vi "Acroname_Port_Enable.vi"(8 "error in (no error)":errorcluster, 9 "Current Max Amps limit (1.2)":dbl=1.2 format="%#_13g", 11 "Port Number":i32) -> (0 "error out":errorcluster, 1 "Max Current (µA)":u32, 2 "Min Voltage (µV)":u32, 3 "Enable Successful?":bool)   [LabVIEW 2025]
uses:
  1b1786e0-183b-4c19-b690-1d9e1fdb2131.vi
  27beaf38-548c-40ef-8c97-2fa24fe30fbd.vi
  31bf49dc-6773-40db-bb53-a572b45535a5.vi
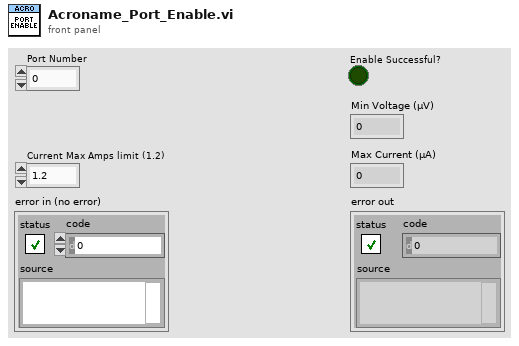
[diagram p1: front panel]
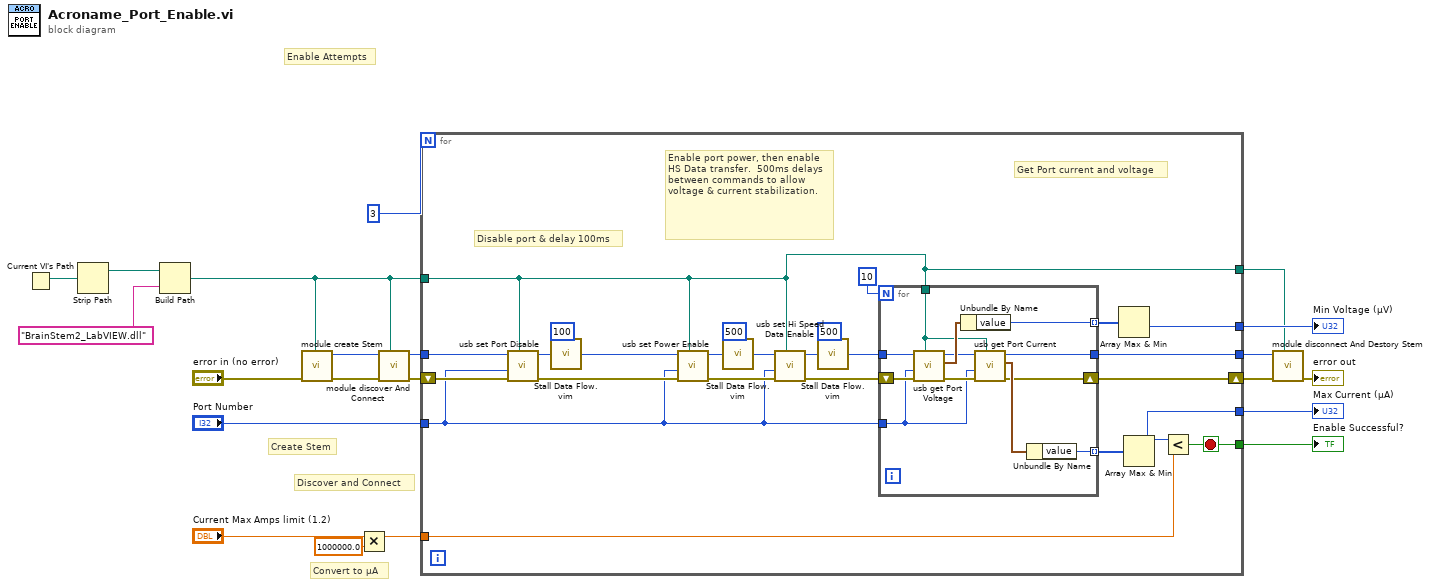
[diagram p0: block diagram]
diagram:
  # "Convert to µA"
  # "Discover and Connect"
  # "Create Stem"
  # "Enable Attempts"
  n1 = Current VI's Path() -> (path=w5:path)
  n2 = Strip Path(path=w5) -> (stripped path=w4:path)  [unwired: 1 out]
  n3 = Build Path(base path=w4, name or relative path="BrainStem2_LabVIEW.dll") -> (appended path=w2:path)
  n4 = call "module create Stem.vi"("dll path in"=w2, "error in (no error)"="error in (no error)") -> ("error out"=w16:errorcluster, "id out"=w21:u32)  [unwired: 7 in, 1 out]
  n5 = Multiply(x="Current Max Amps limit (1.2)", y=1000000.0) -> (x*y=w7:dbl)
  n6 = call "module discover And Connect.vi"("dll path in"=w2, "error in (no error)"=w16, "id"=w21) -> ("error out"=w15:errorcluster, "id out"=w20:u32)  [unwired: 6 in, 1 out]
  n7 = for {
    N: 3 -> [_]
    tunnel: w20 -> [w46]
    tunnel: [w44] -> w19
    tunnel: "Port Number" -> [w30]
    tunnel: w7 -> [w27]
    shift-right: [w26] -> w12
    shift-left: w15 -> [w41]
    tunnel: [w25] -> w10
    tunnel: [w24] -> w9
    tunnel: [w23] -> w8
    tunnel: w2 -> [w22]
    tunnel: [w22] -> w1
    stop <- w25 stop-if-true
    # "Get Port current and voltage"
    # "Enable port power, then enable HS Data transfer.  500ms delays between commands to allow voltage & current stabilization."
    # "Disable port & delay 100ms"
    n8 = call "usb set Port Disable.vi"("dll path in"=w22, "error in (no error)"=w41, "channel"=w30, "id"=w46) -> ("error out"=w39:errorcluster, "id out"=w43:u32)  [unwired: 5 in, 1 out]
    n9 = call "Stall Data Flow.vim"("value in"=w43, "milliseconds to wait"=100) -> ("value out"=w40:u32)  [unwired: 1 out]
    n10 = call "usb set Power Enable.vi"("dll path in"=w22, "error in (no error)"=w39, "channel"=w30, "id"=w40) -> ("error out"=w35:errorcluster, "id out"=w37:u32)  [unwired: 5 in, 1 out]
    n11 = call "Stall Data Flow.vim"("value in"=w37, "milliseconds to wait"=500) -> ("value out"=w36:u32)  [unwired: 1 out]
    n12 = call "usb set Hi Speed Data Enable.vi"("dll path in"=w22, "error in (no error)"=w35, "channel"=w30, "id"=w36) -> ("error out"=w31:errorcluster, "id out"=w33:u32)  [unwired: 5 in, 1 out]
    n13 = call "Stall Data Flow.vim"("value in"=w33, "milliseconds to wait"=500) -> ("value out"=w32:u32)  [unwired: 1 out]
    n14 = for {
      N: 10 -> [_]
      tunnel: w32 -> [w55]
      tunnel: [w54] -> w44
      tunnel: w30 -> [w51]
      shift-right: [w50] -> w26
      shift-left: w31 -> [w53]
      tunnel: [w49] -> w29 mode=indexing
      tunnel: [w48] -> w28 mode=indexing
      tunnel: w22 -> [w47]
      n15 = call "usb get Port Voltage.vi"("dll path in"=w47, "error in (no error)"=w53, "channel"=w51, "id"=w55) -> ("error out"=w52:errorcluster, "result out"=w58:cluster{"value":i32, "error":i32}, "id out"=w56:u32)  [unwired: 5 in]
      n16 = Unbundle By Name(w58) -> ("value"=w49:i32)
      n17 = call "usb get Port Current.vi"("dll path in"=w47, "error in (no error)"=w52, "channel"=w51, "id"=w56) -> ("error out"=w50:errorcluster, "result out"=w57:cluster{"value":i32, "error":i32}, "id out"=w54:u32)  [unwired: 5 in]
      n18 = Unbundle By Name(w57) -> ("value"=w48:i32)
    }
    n19 = Array Max & Min(array=w29) -> (min value=w23:i32)  [unwired: 3 out]
    n20 = Array Max & Min(array=w28) -> (max value=w24:i32)  [unwired: 3 out]
    n21 = Less?(x=w24, y=w27) -> (x < y?=w25:bool)
  }
  "Enable Successful?" <- w10
  "Max Current (µA)" <- w9
  "Min Voltage (µV)" <- w8
  n22 = call "module disconnect And Destory Stem.vi"("dll path in"=w1, "error in (no error)"=w12, "id"=w19) -> ("error out"=→"error out":errorcluster)  [unwired: 6 in, 2 out]
